vi "Motor_Minimal_DC_Stopp.vi"(2 "Turn_off_Trigger_Duty-Cylce":dbl=0.7, 4 "Desired Duty-Cycle":dbl) -> (1 "Triggered Duty-Cycle":dbl)   [LabVIEW 2013]
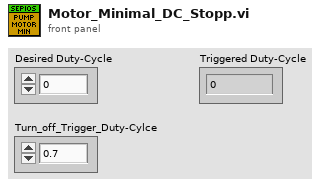
[diagram p1: front panel]
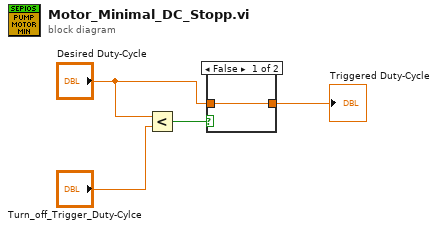
[diagram p0: block diagram]
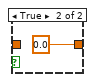
[diagram p2: hidden frame]
diagram:
  n1 = Less?(x="Desired Duty-Cycle", y="Turn_off_Trigger_Duty-Cylce") -> (x < y?=w2:bool)
  n2 = case shown="False" w2 {
    tunnel: [w5 0.0] -> w4
    tunnel: "Desired Duty-Cycle" -> [w5 _]
    frame False {
    }
    frame True {
    }
  }
  "Triggered Duty-Cycle" <- w4
